vi "Z_State_reg.vi"(6 "ZB":bool, 9 "Time":u32[](array[numeric])=[1000, 10000], 10 "Alarm":bool[](array[boolean])=[FALSE, FALSE], 11 "Z_In":cluster{"Z_Source":T1, "Z_SetState":T2}={"Z_Source"=enum."local disabled", "Z_SetState"=enum."alarm"}) -> (1 "t":u32, 3 "Z_Out":cluster{"Z_Source":T1, "Z_State":T2}={"Z_Source"=enum."local disabled", "Z_State"=enum."alarm"}, 4 "N next":u32)   [LabVIEW 2019]
uses:
  Heating/ctl/Y_source.ctl
  Heating/ctl/Z_State.ctl
  Trigers/RS.vi
  Timer Delay/Timer.vi
  Heating/Heating.lvlib
  Userlib.lvlib
panel:
  # "Alarm_L1"
  # "Alarm_L2"
  # "T_stageStop\nT_check\nT_start_delay\nT_heat_start\nT_stop_delay\nT_set_min\nT_heat_stop\nT_restart_delay"
  # "Increase end"
  # "Decrease End"
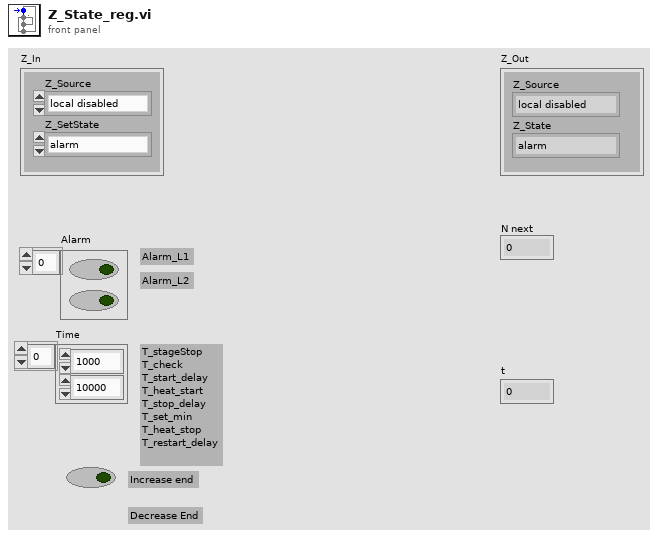
[diagram p1: front panel]
types:
  T1 = typedef "Heating.lvlib/Y_source.ctl" = enum8{"initialize", "local disabled", "local hand", "hand", "auto", "dist"}
  T2 = typedef "Heating.lvlib/Z_State.ctl" = enum8{"initialization", "alarm", "disabled", "not ready", "stop ready", "reserv", "switched off", "reserv2", "switched on", "check", "on min", "decrease out", "on", "increase out", "on max"}
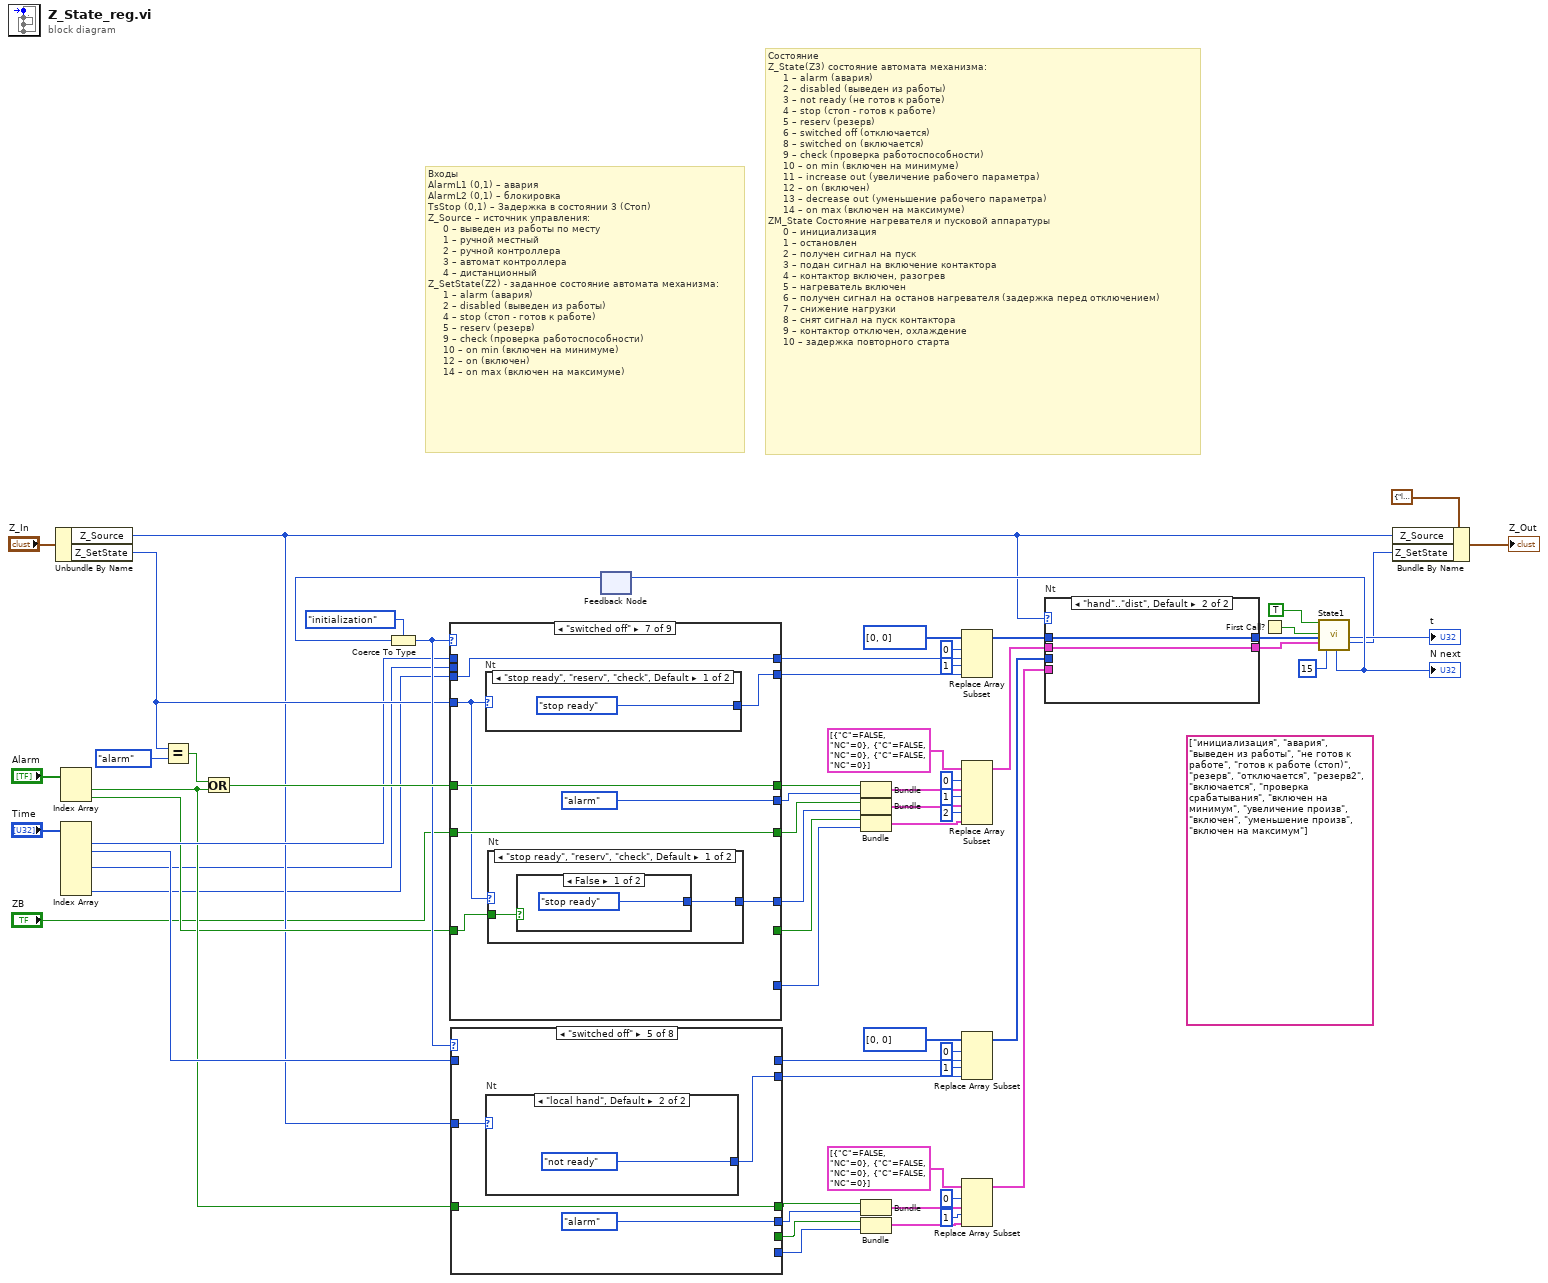
[diagram p0: block diagram]
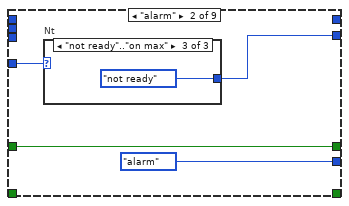
[diagram p4: hidden frame]
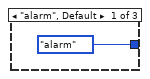
[diagram p5: hidden frame]
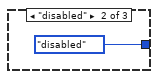
[diagram p6: hidden frame]
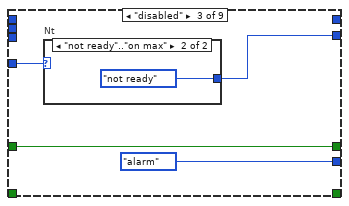
[diagram p7: hidden frame]
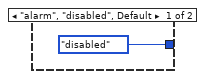
[diagram p8: hidden frame]
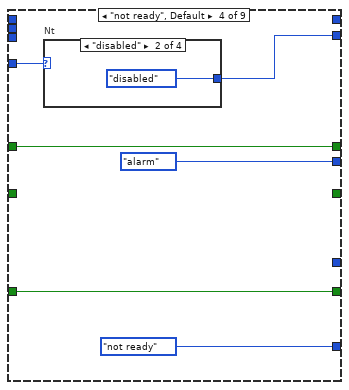
[diagram p9: hidden frame]
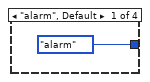
[diagram p10: hidden frame]
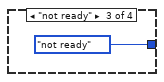
[diagram p11: hidden frame]
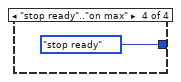
[diagram p12: hidden frame]
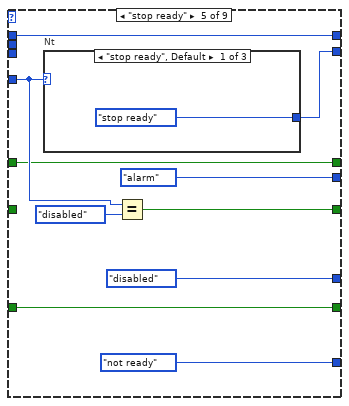
[diagram p13: hidden frame]
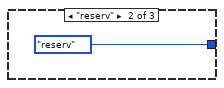
[diagram p14: hidden frame]
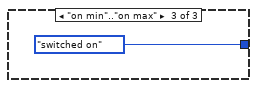
[diagram p15: hidden frame]
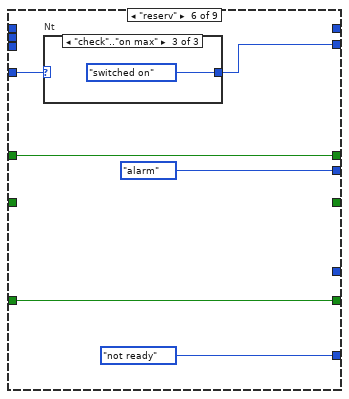
[diagram p16: hidden frame]
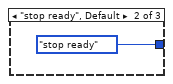
[diagram p18: hidden frame]
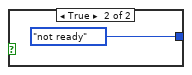
[diagram p19: hidden frame]
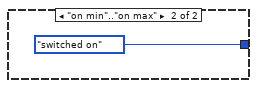
[diagram p20: hidden frame]
diagram:
  (unwired) string[] ["инициализация", "авария", "выведен из работы", "не готов к работе", "готов к работе (стоп)", "резерв", "отключается", "резерв2", "включается", "проверка срабатывания", "включен на минимум", "увеличение произв", "включен", "уменьшение произв", "включен на максимум"]
  # "Входы\nAlarmL1 (0,1) – авария\nAlarmL2 (0,1) – блокировка\nTsStop (0,1) – Задержка в состоянии 3 (Стоп)\nZ_Source – источник управления:\n     0 – выведен из работы по месту\n     1 – ручной местный\n     2 – ручной контроллера\n     3 – автомат контроллера\n     4 – дистанционный\nZ_SetState(Z2) - заданное состояние автомата механизма:\n     1 – alarm (авария)\n     2 – disabled (выведен из работы)\n     4 – stop (стоп - готов к работе)\n     5 – reserv (резерв)\n     9 – check (проверка работоспособности)\n     10 – on min (включен на минимуме)\n     12 – on (включен)\n     14 – on max (включен на максимуме)"
  # "Состояние\nZ_State(Z3) состояние автомата механизма:\n     1 – alarm (авария)\n     2 – disabled (выведен из работы)\n     3 – not ready (не готов к работе)\n     4 – stop (стоп - готов к работе)\n     5 – reserv (резерв)\n     6 – switched off (отключается)\n     8 – switched on (включается)\n     9 – check (проверка работоспособности)\n     10 – on min (включен на минимуме)\n     11 – increase out (увеличение рабочего параметра)\n     12 – on (включен)\n     13 – decrease out (уменьшение рабочего параметра)\n     14 – on max (включен на максимуме)\nZM_State Состояние нагревателя и пусковой аппаратуры\n     0 – инициализация\n     1 – остановлен\n     2 – получен сигнал на пуск\n     3 – подан сигнал на включение контактора\n     4 – контактор включен, разогрев\n     5 – нагреватель включен\n     6 – получен сигнал на останов нагревателя (задержка перед отключением)\n     7 – снижение нагрузки\n     8 – снят сигнал на пуск контактора\n     9 – контактор отключен, охлаждение\n     10 – задержка повторного старта"
  n1 = Unbundle By Name("Z_In") -> ("Z_Source"=w4:T1, "Z_SetState"=w58:T2)
  n2 = Index Array(array="Alarm") -> (element #1=w50:bool, element #2=w49:bool)  [unwired: 2 in]
  n3 = Index Array(array="Time") -> (element #1=w53:u32, element #2=w52:u32, element #4=w2:u32, element #7=w1:u32)  [unwired: 7 in, 3 out]
  n4 = Equal?(x=w58, y=Z_State."alarm") -> (x = y?=w64:bool)
  n5 = Or(x=w64, y=w50) -> (x .or. y?=w63:bool)
  n6 = feedback #1() -> (w60:u32)  [unwired: 1 in]
  n7 = Coerce To Type(0:w60, 1:Z_State."initialization" ("Z_SetState")) -> (2:w59:T2)
  n8 = case shown="\"switched off\"" w59 {
    tunnel: w63 -> [_ w68 w75 w83 w93 w106 w118 w135 w149]
    tunnel: w58 -> [w65 w69 w76 w84 w97 w107 w113 w126 w145]
    tunnel: w49 -> [_ _ _ w81 w95 w105 w111 w129 w147]
    tunnel: w53 -> [_ _ _ _ w96 _ _ _ _]
    tunnel: [_ _ _ Z_State."not ready" ("Z_SetState") Z_State."not ready" ("Z_SetState") Z_State."not ready" ("Z_SetState") _ Z_State."switched off" ("Z_SetState") Z_State."switched off" ("Z_SetState")] -> w12
    tunnel: [_ _ _ _ w96 _ w115 w132 _] -> w18
    tunnel: [_ _ _ w81 w95 w105 _ w136 w148] -> w11
    tunnel: [_ _ _ _ Z_State."disabled" ("Z_SetState") _ w112 w127 _] -> w10
    tunnel: [_ _ _ _ w94 _ w114 w128 _] -> w13
    tunnel: [_ Z_State."alarm" ("Z_SetState") Z_State."alarm" ("Z_SetState") Z_State."alarm" ("Z_SetState") Z_State."alarm" ("Z_SetState") Z_State."alarm" ("Z_SetState") Z_State."alarm" ("Z_SetState") Z_State."alarm" ("Z_SetState") Z_State."alarm" ("Z_SetState")] -> w14
    tunnel: [_ w68 w75 w83 w93 w106 w118 w135 w149] -> w15
    tunnel: [w65 w67 w74 w82 w92 w104 w117 w131 w145] -> w17
    tunnel: "ZB" -> [_ _ _ _ _ _ w114 w128 _]
    tunnel: w1 -> [_ _ _ _ _ _ w115 _ _]
    tunnel: w2 -> [_ _ _ _ _ _ _ w132 _]
    frame "initialization" {
    }
    frame "alarm" {
      n9 = case "Nt" shown="\"not ready\"..\"on max\"" w69 {
        tunnel: [Z_State."alarm" ("Z_SetState") Z_State."disabled" ("Z_SetState") Z_State."not ready" ("Z_SetState")] -> w67
        frame "alarm", Default {
        }
        frame "disabled" {
        }
        frame "not ready".."on max" {
        }
      }
    }
    frame "disabled" {
      n10 = case "Nt" shown="\"not ready\"..\"on max\"" w76 {
        tunnel: [Z_State."disabled" ("Z_SetState") Z_State."not ready" ("Z_SetState")] -> w74
        frame "alarm", "disabled", Default {
        }
        frame "not ready".."on max" {
        }
      }
    }
    frame "not ready", Default {
      n11 = case "Nt" shown="\"disabled\"" w84 {
        tunnel: [Z_State."alarm" ("Z_SetState") Z_State."disabled" ("Z_SetState") Z_State."not ready" ("Z_SetState") Z_State."stop ready" ("Z_SetState")] -> w82
        frame "alarm", Default {
        }
        frame "disabled" {
        }
        frame "not ready" {
        }
        frame "stop ready".."on max" {
        }
      }
    }
    frame "stop ready" {
      n12 = case "Nt" shown="\"stop ready\", Default" w97 {
        tunnel: [Z_State."stop ready" ("Z_SetState") Z_State."reserv" ("Z_SetState") Z_State."switched on" ("Z_SetState")] -> w92
        frame "stop ready", Default {
        }
        frame "reserv" {
        }
        frame "on min".."on max" {
        }
      }
      n13 = Equal?(x=w97, y=Z_State."disabled") -> (x = y?=w94:bool)
    }
    frame "reserv" {
      n14 = case "Nt" shown="\"check\"..\"on max\"" w107 {
        selector: w107 -> [w108 _ _]
        tunnel: [w108 Z_State."stop ready" ("Z_SetState") Z_State."switched on" ("Z_SetState")] -> w104
        frame "alarm".."not ready", "reserv" {
        }
        frame "stop ready", Default {
        }
        frame "check".."on max" {
        }
      }
    }
    frame "switched off" {
      n15 = case "Nt" shown="\"stop ready\", \"reserv\", \"check\", Default" w113 {
        tunnel: [Z_State."stop ready" ("Z_SetState") Z_State."switched on" ("Z_SetState")] -> w117
        frame "stop ready", "reserv", "check", Default {
        }
        frame "on min".."on max" {
        }
      }
      n16 = case "Nt" shown="\"stop ready\", \"reserv\", \"check\", Default" w113 {
        tunnel: [w120 Z_State."switched on" ("Z_SetState")] -> w112
        tunnel: w111 -> [w119 _]
        frame "stop ready", "reserv", "check", Default {
          n17 = case shown="False" w119 {
            tunnel: [Z_State."stop ready" ("Z_SetState") Z_State."not ready" ("Z_SetState")] -> w120
            frame False {
            }
            frame True {
            }
          }
        }
        frame "on min".."on max" {
        }
      }
    }
    frame "switched on" {
      n18 = case "Nt" shown="\"stop ready\", \"reserv\", \"check\", Default" w126 {
        selector: w126 -> [_ w140]
        tunnel: [Z_State."switched off" ("Z_SetState") w140] -> w131
        frame "stop ready", "reserv", "check", Default {
        }
        frame "on min".."on max" {
        }
      }
      n19 = case "Nt" shown="\"stop ready\", \"reserv\", \"check\", Default" w126 {
        selector: w126 -> [_ w138]
        tunnel: [Z_State."switched off" ("Z_SetState") w138] -> w127
        frame "stop ready", "reserv", "check", Default {
        }
        frame "on min".."on max" {
        }
      }
      n20 = case "Z2" shown="\"disabled\"..\"reserv\", Default" w126 {
        tunnel: [FALSE TRUE] -> w130
        frame "check".."on max" {
        }
        frame "disabled".."reserv", Default {
        }
      }
      n21 = Or(x=w129, y=w130) -> (x .or. y?=w136:bool)
    }
    frame "check".."on max" {
      n22 = case "Z2" shown="\"disabled\"..\"reserv\", Default" w145 {
        tunnel: [FALSE TRUE] -> w146
        frame "check".."on max" {
        }
        frame "disabled".."reserv", Default {
        }
      }
      n23 = Or(x=w146, y=w147) -> (x .or. y?=w148:bool)
    }
  }
  n24 = case shown="\"switched off\"" w59 {
    tunnel: w50 -> [_ w156 _ w166 w172 w177 w182 w185]
    tunnel: w4 -> [_ w155 w160 w165 w171 _ _ _]
    tunnel: [_ _ _ _ _ _ w181 _] -> w5
    tunnel: [_ _ _ _ _ _ FALSE _] -> w6
    tunnel: [_ Z_State."alarm" ("Z_SetState") _ Z_State."alarm" ("Z_SetState") Z_State."alarm" ("Z_SetState") Z_State."alarm" ("Z_SetState") Z_State."alarm" ("Z_SetState") Z_State."alarm" ("Z_SetState")] -> w7
    tunnel: [_ w156 _ w166 w172 w177 w182 w185] -> w8
    tunnel: [Z_State."not ready" ("Z_SetState") w154 w159 w164 w170 Z_State."not ready" ("Z_SetState") w181 Z_State."on" ("Z_SetState")] -> w9
    tunnel: w52 -> [_ _ _ _ _ _ w179 _]
    tunnel: [_ _ _ _ _ _ w179 _] -> w16
    frame "initialization" {
    }
    frame "alarm" {
      n25 = case "Nt" shown="\"local hand\"" w155 {
        tunnel: [Z_State."disabled" ("Z_SetState") Z_State."not ready" ("Z_SetState")] -> w154
        frame "local disabled", Default {
        }
        frame "local hand" {
        }
      }
    }
    frame "disabled", "stop ready", "reserv", "reserv2" {
      n26 = case "Nt" shown="\"local disabled\", Default" w160 {
        tunnel: [Z_State."disabled" ("Z_SetState") Z_State."not ready" ("Z_SetState")] -> w159
        frame "local disabled", Default {
        }
        frame "local hand" {
        }
      }
    }
    frame "not ready", Default {
      n27 = case "Nt" shown="\"local disabled\", Default" w165 {
        tunnel: [Z_State."disabled" ("Z_SetState") Z_State."not ready" ("Z_SetState")] -> w164
        frame "local disabled", Default {
        }
        frame "local hand" {
        }
      }
    }
    frame "switched off" {
      n28 = case "Nt" shown="\"local hand\", Default" w171 {
        tunnel: [Z_State."disabled" ("Z_SetState") Z_State."not ready" ("Z_SetState")] -> w170
        frame "local disabled" {
        }
        frame "local hand", Default {
        }
      }
    }
    frame "switched on" {
    }
    frame "check" {
      w181 = Z_State."on" ("Z_SetState")
    }
    frame "on min".."on max" {
    }
  }
  n29 = Bundle(w15, "Z_SetState"=w14) -> (w40:cluster{bool, "Z_SetState":T2})  [unwired: 1 in]
  n30 = Bundle("ZB"=w13, "Z_SetState"=w10) -> (w37:cluster{"ZB":bool, "Z_SetState":T2})  [unwired: 1 in]
  n31 = Bundle("Alarm"=w11, "Z_SetState"=w12) -> (w36:cluster{"Alarm":bool, "Z_SetState":T2})  [unwired: 1 in]
  n32 = Bundle("Alarm"=w8, "Z_SetState"=w7) -> (w33:cluster{"Alarm":bool, "Z_SetState":T2})  [unwired: 1 in]
  n33 = Bundle(w6, "Z_SetState"=w5) -> (w35:cluster{bool, "Z_SetState":T2})  [unwired: 1 in]
  n34 = Replace Array Subset(array=u32[] [0, 0] ("appended array"), new element #1=w18, index #1=0 ("index"), new element #2=w17, index #2=1 ("index")) -> (w25:u32[])
  n35 = Replace Array Subset(array=cluster{"C":bool, "NC":u32}[] [{"C"=FALSE, "NC"=0}, {"C"=FALSE, "NC"=0}, {"C"=FALSE, "NC"=0}] ("appended array"), new element #1=w40, index #1=0 ("index"), new element #2=w37, index #2=1 ("index"), new element #3=w36, index #3=2 ("index")) -> (w23:cluster{"C":bool, "NC":u32}[])
  n36 = Replace Array Subset(array=u32[] [0, 0] ("appended array"), new element #1=w16, index #1=0 ("index"), new element #2=w9, index #2=1 ("index")) -> (w27:u32[])
  n37 = Replace Array Subset(array=cluster{"C":bool, "NC":u32}[] [{"C"=FALSE, "NC"=0}, {"C"=FALSE, "NC"=0}, {"C"=FALSE, "NC"=0}] ("appended array"), new element #1=w33, index #1=0 ("index"), new element #2=w35, index #2=1 ("index")) -> (w26:cluster{"C":bool, "NC":u32}[])
  n38 = case "Nt" shown="\"hand\"..\"dist\", Default" w4 {
    tunnel: w25 -> [_ w189]
    tunnel: w23 -> [_ w188]
    tunnel: [w186 w189] -> w24
    tunnel: [w187 w188] -> w22
    tunnel: w27 -> [w186 _]
    tunnel: w26 -> [w187 _]
    frame "local disabled", "local hand" {
    }
    frame "hand".."dist", Default {
    }
  }
  n39 = First Call?() -> (First Call?: T/F=w47:bool)
  n40 = call "State1.vi"("Start"=TRUE, "Reset"=w47, "T_table"=w24, "C_table"=w22, "End step"=u32 15) -> ("N next"=w21:u32, "t"=→"t":u32, "N curr"=w19:u32)  [unwired: 9 in, 3 out]
  "N next" <- w21
  n41 = feedback-in #1(w21) -> ()
  n42 = Bundle By Name(cluster=cluster{"Z_Source":T1, "Z_SetState":T2} {"Z_Source"=enum."local disabled", "Z_SetState"=enum."alarm"} ("Z_Out"), "Z_Source"=w4, "Z_SetState"=w19) -> (→"Z_Out":cluster{"Z_Source":T1, "Z_SetState":T2})
